vi "Decoration - Image.vi"() -> ()   [LabVIEW 2017]
doc: "Sample numeric display item."
uses:
  <vilib>/NI Veristand/Display Template Support/Display Template Support.llb/cluster_Screen Item Settings.ctl
  <vilib>/NI Veristand/Display Template Support/Display Template Support.llb/cluster_Graph Scale Settings.ctl
  <vilib>/NI Veristand/Display Template Support/Display Template Support.llb/cluster_Graph Plot Settings.ctl
  <vilib>/NI Veristand/Display Template Support/Display Template Support.llb/enum_Display Template Handler Minimal To Widget Msg.ctl
  <vilib>/NI Veristand/Display Template Support/Display Template Support.llb/enum_Display Template Handler Minimal To Workspace.ctl
  Picture Configuration.ctl
  <vilib>/NI Veristand/Display Template Support/Display Template Support.llb/sub_Display Template Handler Custom.vi
panel:
  out "Image":picture
  in  "Item.Data":T1
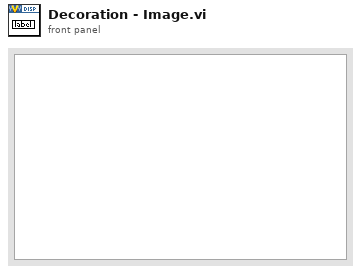
[diagram p1: front panel]
types:
  T1 = typedef "cluster_Screen Item Settings.ctl" = cluster{"Template VI":string, "Position X":i32, "Position Y":i32, "Custom":string, "Show Title Bar":bool, "ID":i32, "Always On Top":bool, "Allow Resize":bool, "Allow Minimize":bool, "Allow Close":bool, "Size to Screen":bool, "Screen.ID":i32, "State":enum16{"Normal", "New"}, "Title":string, "Window Bounds":cluster{"[0]":i16, "[1]":i16, "[2]":i16, "[3]":i16}, "Channel Ref":u64, "Unit":string, "Default Units?":bool, "Flash Limit?":bool, "Color 1":u32, "Color 2":u32, "Color 3":u32, "Color 4":u32, "Bck Color":u32, "Fore Color":u32, "Limit 1":dbl, "Limit 2":dbl, "Limit 3":dbl, "Limit 4":dbl, "Limit Mode 1":i32, "Limit Mode 2":i32, "Limit Mode 3":i32, "Limit Mode 4":i32, "Scale Precision":i32, "Scale Min":dbl, "Scale Max":dbl, "Format":i32, "Precision":i32, "Background Type":i32, "IDs":i32[], "Units":string[], "Labels":string[], "Scale Factor":dbl, "Scale Offset":dbl, "YScale Index":u32[], "XScale":T2, "YScales":T2[], "Plots":T3[], "Update Period":dbl, "History Length":dbl, "My.Ref":refnum<vi>, "Is Control?":bool, "Channel Paths":string[], "Custom Data":variant}
  T2 = typedef "cluster_Graph Scale Settings.ctl" = cluster{"Format":u8, "Precision":u8, "Fit":u8, "Label":string, "Use Default Label":bool, "Label Visible":bool, "Min":dbl, "Max":dbl}
  T3 = typedef "cluster_Graph Plot Settings.ctl" = cluster{"Bar Style":u8, "Fill To":i16, "Fill/PtColor":u32, "Line Style":u8, "Line Width":u8, "Color":u32, "Interp":u8, "Point Style":u8}
  T4 = typedef "enum_Display Template Handler Minimal To Workspace.ctl" = cluster{"Operation":enum16{"SetCustomData", "DeleteItem"}, "Data":variant}
  T5 = typedef "enum_Display Template Handler Minimal To Widget Msg.ctl" = enum16{"Stop", "LaunchConfigDialog"}
  T6 = typedef "Picture Configuration.ctl" = cluster{"Path":path, "Start Pixels":cluster{"X":i32, "Y":i32}, "Rotation":dbl, "Rotation Pixels":cluster{"X":i32, "Y":i32}, "Scale":dbl}
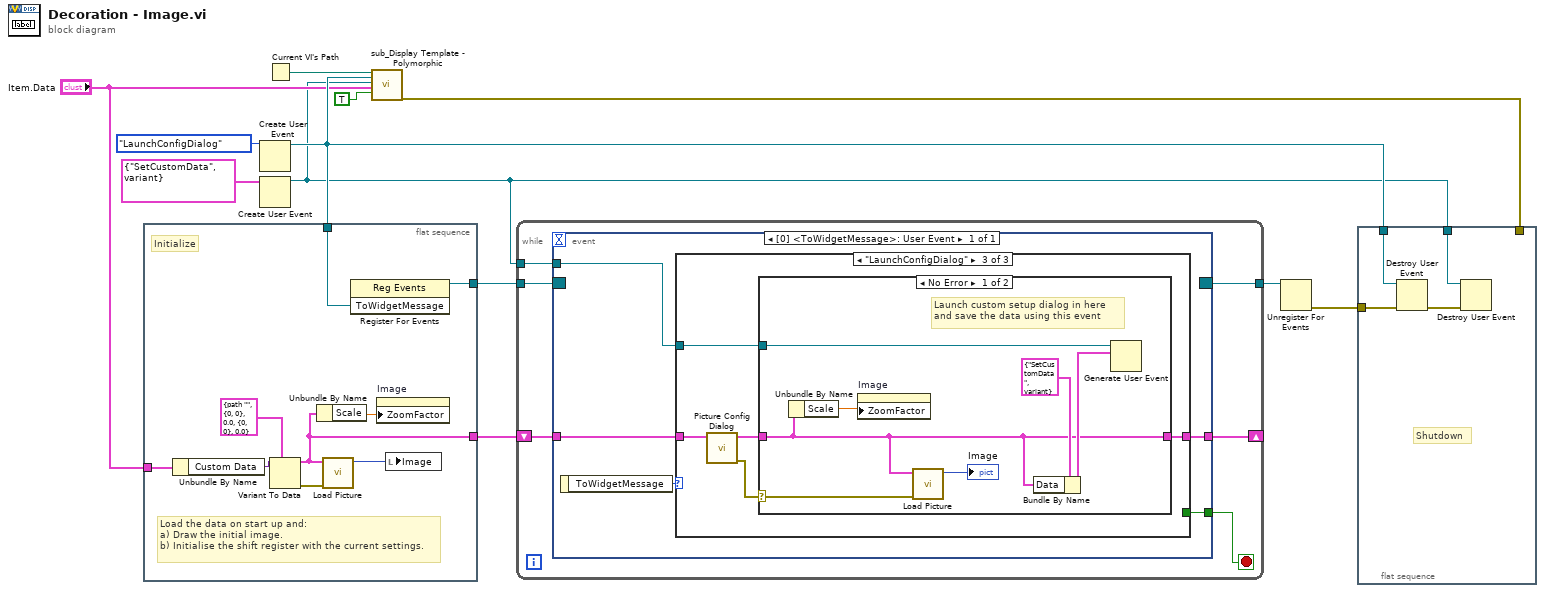
[diagram p0: block diagram]
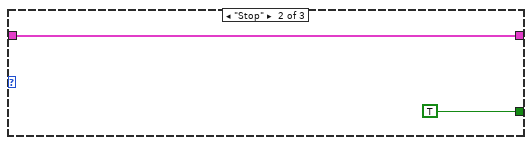
[diagram p3: hidden frame]
diagram:
  n1 = flat-sequence {
    tunnel: [w21] -> w10
    tunnel: w7 -> [w20]
    tunnel: "Item.Data" -> [w19]
    tunnel: [w14] -> w1
    frame #0 {
      # "Load the data on start up and:\na) Draw the initial image.\nb) Initialise the shift register with the current settings."
      # "Initialize"
      n2 = Unbundle By Name(w19) -> ("Custom Data"=w18:variant)
      n3 = Variant To Data(type=T6 {"Path"=path "", "Start Pixels"={"X"=0, "Y"=0}, "Rotation"=0.0, "Rotation Pixels"={"X"=0, "Y"=0}, "Scale"=0.0} ("Picture Config Out"), Variant=w18) -> (data=w14:T6, error out=w17:errorcluster)  [unwired: 1 in]
      n4 = Unbundle By Name(w14) -> ("Scale"=w13:dbl)
      n5 = call "Load Picture.vi"("error in (no error)"=w17, "Picture Config"=w14) -> ("Picture from File"=w16:picture)  [unwired: 8 in, 1 out]
      n6 = register-events(w20) -> (reference out=w21:refnum<event-registration>)  [unwired: 2 in, 1 out]
      n7 = property on="Image" class="Pict"("ZoomFactor"=w13) -> ()  [unwired: 2 in, 2 out]
      n8 = local write "Image"(w16) -> ()
    }
  }
  n9 = Create User Event(user event datatype=enum_Display_Template_Handler_Minimal_To_Widget_Msg."LaunchConfigDialog" ("ToWidgetMessage")) -> (user event=w7:refnum<user-event>)  [unwired: 1 in, 1 out]
  n10 = Create User Event(user event datatype=T4 {"Operation"=enum."SetCustomData", "Data"=variant} ("Data")) -> (user event=w3:refnum<user-event>)  [unwired: 1 in, 1 out]
  n11 = Current VI's Path() -> (path=w5:path)
  n12 = call-poly <vilib>:"sub_Display Template - Polymorphic.vi"("Parent.Path"=w5, "ToWidgetEvent"=w7, "ToWorkspace"=w3, "Item.Data"="Item.Data", "Resizable"=TRUE) -> ("error out"=w12:errorcluster)  [unwired: 1 in, 13 out]
  n13 = while {
    tunnel: w10 -> [w27]
    tunnel: [w25] -> w9
    tunnel: w3 -> [w24]
    shift-right: [w23] -> _
    shift-left: w1 -> [w22]
    stop <- w26 stop-if-true
    n14 = event shown="[0] <ToWidgetMessage>: User Event" {
      selector: w27 -> [_]
      dyn-events: [_] -> w25
      timeout: _ -> [_]
      tunnel: [w31] -> w26
      tunnel: w24 -> [w30]
      tunnel: [w29] -> w23
      tunnel: w22 -> [w28]
      event User Event {
        n15 = event-data() -> ("ToWidgetMessage"=w32:T5)  [unwired: 1 out]
        n16 = case shown="\"LaunchConfigDialog\"" w32 {
          tunnel: [_ TRUE _] -> w31
          tunnel: w30 -> [_ _ w40]
          tunnel: [w33 w34 w37] -> w29
          tunnel: w28 -> [w33 w34 w36]
          frame Default {
          }
          frame "Stop" {
          }
          frame "LaunchConfigDialog" {
            n17 = call "Picture Config Dialog.vi"("Picture Config In"=w36) -> ("error out"=w38:errorcluster, "Picture Config Out"=w39:T6)  [unwired: 9 in]
            n18 = case shown="No Error" w38 {
              selector: w38 -> [w43 _]
              tunnel: w40 -> [w47 _]
              tunnel: w39 -> [w42 w48]
              tunnel: [w42 w48] -> w37
              frame No Error {
                # "Launch custom setup dialog in here\nand save the data using this event"
                n19 = Unbundle By Name(w42) -> ("Scale"=w41:dbl)
                n20 = property on="Image" class="Pict"("ZoomFactor"=w41) -> ()  [unwired: 2 in, 2 out]
                n21 = call "Load Picture.vi"("error in (no error)"=w43, "Picture Config"=w42) -> ("Picture from File"=→"Image":picture)  [unwired: 8 in, 1 out]
                n22 = Bundle By Name(cluster=T4 {"Operation"=enum."SetCustomData", "Data"=variant} ("event data"), "Data"=w42) -> (w45:T4)
                n23 = Generate User Event(user event=w47, event data cluster=w45) -> ()  [unwired: 2 in, 2 out]
              }
              frame Error {
              }
            }
          }
        }
      }
    }
  }
  n24 = Unregister For Events(event registration refnum=w9) -> (error out=w8:errorcluster)  [unwired: 1 in]
  n25 = flat-sequence {
    tunnel: w12 -> [_]
    tunnel: w8 -> [w51]
    tunnel: w7 -> [w52]
    tunnel: w3 -> [w49]
    frame #0 {
      # "Shutdown"
      n26 = Destroy User Event(user event=w52, error in=w51) -> (error out=w50:errorcluster)
      n27 = Destroy User Event(user event=w49, error in=w50) -> ()  [unwired: 1 out]
    }
  }
